vi "参数设置2.0.vi"(0 "速度(Hz)":dbl=3000.0, 1 "导程":dbl=4.0, 2 "速度(Hz)":dbl=3000.0, 3 "导程":dbl=4.0, 4 "速度(Hz)":dbl=3000.0, 5 "导程":dbl=5.0, 6 "回零速度":dbl=8400.0, 7 "精度":dbl=0.001, 8 "数据小数位":dbl=12.0) -> (11 "数据小数位":dbl=12.0, 12 "回零速度":dbl, 13 "精度":dbl, 14 "速度(Hz) 2":dbl, 15 "导程 2":dbl, 16 "速度(Hz)  3":dbl, 17 "导程 3":dbl, 18 "速度(Hz) 3":dbl, 19 "导程 4":dbl)   [LabVIEW 2016]
panel:
  in  "空白按钮":bool
  # "参数设置"
  # "X"
  # "Y"
  # "Z"
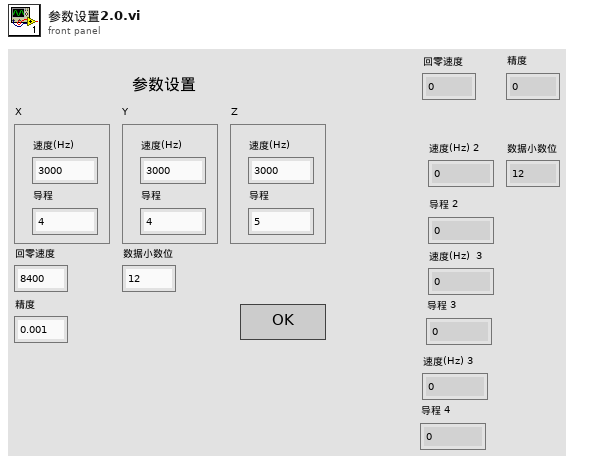
[diagram p1: front panel]
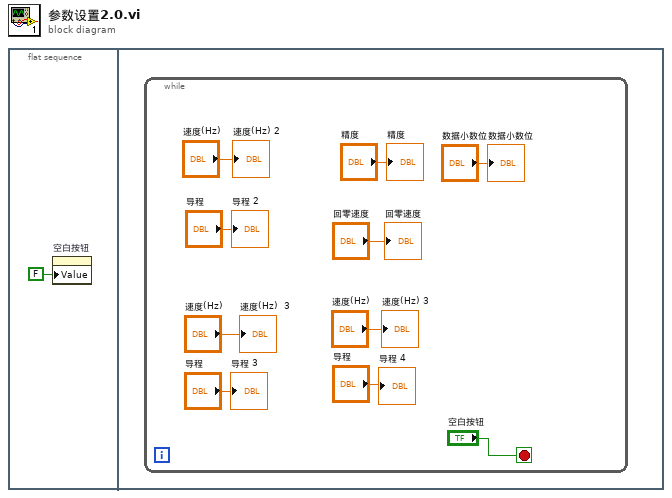
[diagram p0: block diagram]
diagram:
  n1 = flat-sequence {
    frame #0 {
      n2 = property on="空白按钮" class="Bool (严格)"("Value"=FALSE ("空白按钮")) -> ()  [unwired: 2 in, 2 out]
    }
    frame #1 {
      n3 = while {
        stop <- "空白按钮" stop-if-true
        "导程 2" <- "导程"
        "速度(Hz) 2" <- "速度(Hz)"
        "精度" <- "精度"
        "回零速度" <- "回零速度"
        "速度(Hz)  3" <- "速度(Hz)"
        "导程 3" <- "导程"
        "速度(Hz) 3" <- "速度(Hz)"
        "导程 4" <- "导程"
        "数据小数位" <- "数据小数位"
      }
    }
  }
